vi "N5232-PNA_ReadChanTrigger.vi"(0 "Session In":refnum<visa-resource-name>="TCPIP0::169.254.70.180::inst0::INSTR", 5 "CHANNEL":i32=1, 11 "error in":errorcluster {"code" format="%.0x"}) -> (4 "Session Out":refnum<visa-resource-name>, 6 "SWE-MODE?":string, 8 "GROUP-COUNT":string, 10 "TRG-MODE":string, 15 "error out":errorcluster {"code" format="%.0x"})   [LabVIEW 2018]
doc: "Launches the Instrument I/O Assistant, which you can use to communicate with message-based instruments and graphically parse the response. For example you can communicate with an instrument that uses a serial, Ethernet, or GPIB interface."
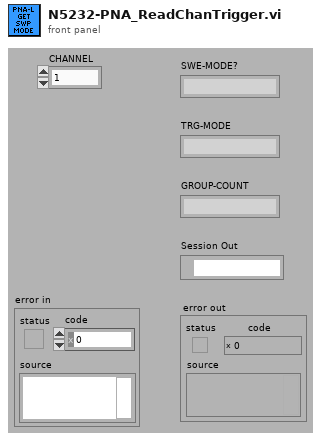
[diagram p1: front panel]
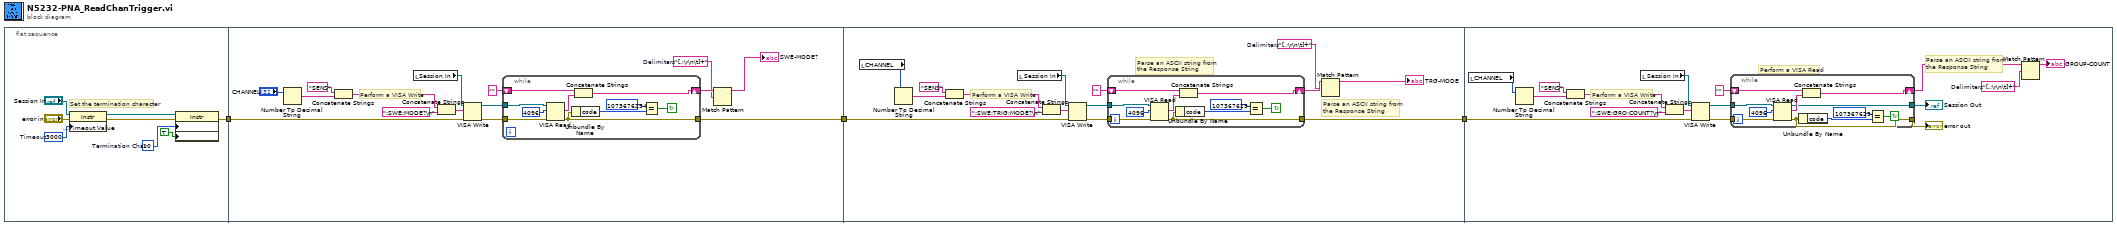
[diagram p0: block diagram]
diagram:
  n1 = flat-sequence {
    tunnel: [w7] -> w3
    tunnel: w3 -> [w17]
    tunnel: [w15] -> w2
    tunnel: w2 -> [w42]
    tunnel: [w40] -> w1
    tunnel: w1 -> [w67]
    frame #0 {
      w6 = u8 10  # Termination Char
      w10 = u32 3000  # Timeout
      # "Set the termination character"
      n2 = property class="Instr"(reference="Session In", error in="error in", "General Settings:Timeout Value"=w10) -> (reference out=w5:refnum<visa-resource-name>, error out=w8:errorcluster)
      n3 = property class="Instr"(reference=w5, error in=w8, "Message Based Settings:Termination Character"=w6, "Message Based Settings:Termination Character Enable"=TRUE ("enable")) -> (error out=w7:errorcluster)  [unwired: 1 in]
    }
    frame #1 {
      w20 = "[,;\r\n\t]+"  # Delimiters
      # "Perform a VISA Write"
      n4 = Number To Decimal String(number="CHANNEL") -> (decimal integer string=w22:string)  [unwired: 1 out]
      n5 = Concatenate Strings("SENS" ("staticText"), w22) -> (w25:string)
      n6 = local read "Session In"() -> (w14:refnum<visa-resource-name>)
      n7 = Concatenate Strings(w25, ":SWE:MODE?\n" ("StaticText")) -> (w24:string)
      n8 = VISA Write(VISA resource name=w14, write buffer=w24, error in (no error)=w17) -> (VISA resource name out=w13:refnum<visa-resource-name>, error out=w23:errorcluster)  [unwired: 1 out]
      n9 = while {
        tunnel: w13 -> [w27]
        shift-left: "" -> [w30]
        shift-right: [w29] -> w26
        tunnel: w23 -> [w28]
        tunnel: [w32] -> w15
        stop <- w34 continue-if-true
        n10 = VISA Read(VISA resource name=w27, byte count=u32 4096 ("byte count (0)"), error in (no error)=w28) -> (read buffer=w31:string, error out=w32:errorcluster)  [unwired: 2 out]
        n11 = Unbundle By Name(w32) -> ("code"=w35:i32)
        n12 = Concatenate Strings(w30, w31) -> (w29:string)
        n13 = Equal?(x=1073676294, y=w35) -> (x = y?=w34:bool)
      }
      n14 = Match Pattern(string=w26, regular expression=w20) -> (before substring=→"SWE-MODE?":string)  [unwired: 4 out]
    }
    frame #2 {
      w45 = "[,;\r\n\t]+"  # Delimiters
      # "Parse an ASCII string from the Response String"
      # "Perform a VISA Write"
      # "Parse an ASCII string from the Response String"
      n15 = local read "CHANNEL"() -> (w37:i32)
      n16 = Number To Decimal String(number=w37) -> (decimal integer string=w46:string)  [unwired: 1 out]
      n17 = Concatenate Strings("SENS" ("staticText"), w46) -> (w49:string)
      n18 = local read "Session In"() -> (w38:refnum<visa-resource-name>)
      n19 = Concatenate Strings(w49, ":SWE:TRIG:MODE?\n" ("StaticText")) -> (w48:string)
      n20 = VISA Write(VISA resource name=w38, write buffer=w48, error in (no error)=w42) -> (VISA resource name out=w39:refnum<visa-resource-name>, error out=w47:errorcluster)  [unwired: 1 out]
      n21 = while {
        shift-left: "" -> [w55]
        shift-right: [w54] -> w51
        tunnel: w47 -> [w53]
        tunnel: [w57] -> w40
        tunnel: w39 -> [w52]
        stop <- w59 continue-if-true
        n22 = VISA Read(VISA resource name=w52, byte count=u32 4096 ("byte count (0)"), error in (no error)=w53) -> (read buffer=w56:string, error out=w57:errorcluster)  [unwired: 2 out]
        n23 = Unbundle By Name(w57) -> ("code"=w60:i32)
        n24 = Concatenate Strings(w55, w56) -> (w54:string)
        n25 = Equal?(x=1073676294, y=w60) -> (x = y?=w59:bool)
      }
      n26 = Match Pattern(string=w51, regular expression=w45) -> (before substring=→"TRG-MODE":string)  [unwired: 4 out]
    }
    frame #3 {
      w70 = "[,;\r\n\t]+"  # Delimiters
      # "Parse an ASCII string from the Response String"
      # "Perform a VISA Read"
      # "Perform a VISA Write"
      n27 = local read "CHANNEL"() -> (w62:i32)
      n28 = Number To Decimal String(number=w62) -> (decimal integer string=w71:string)  [unwired: 1 out]
      n29 = Concatenate Strings("SENS" ("staticText"), w71) -> (w74:string)
      n30 = local read "Session In"() -> (w65:refnum<visa-resource-name>)
      n31 = Concatenate Strings(w74, ":SWE:GRO:COUNT?\n" ("StaticText")) -> (w73:string)
      n32 = VISA Write(VISA resource name=w65, write buffer=w73, error in (no error)=w67) -> (VISA resource name out=w64:refnum<visa-resource-name>, error out=w72:errorcluster)  [unwired: 1 out]
      n33 = while {
        shift-left: "" -> [w82]
        shift-right: [w81] -> w77
        tunnel: w72 -> [w80]
        tunnel: [w84] -> w75
        tunnel: w64 -> [w79]
        tunnel: [w78] -> w63
        stop <- w86 continue-if-true
        n34 = VISA Read(VISA resource name=w79, byte count=u32 4096 ("byte count (0)"), error in (no error)=w80) -> (VISA resource name out=w78:refnum<visa-resource-name>, read buffer=w83:string, error out=w84:errorcluster)  [unwired: 1 out]
        n35 = Unbundle By Name(w84) -> ("code"=w87:i32)
        n36 = Concatenate Strings(w82, w83) -> (w81:string)
        n37 = Equal?(x=1073676294, y=w87) -> (x = y?=w86:bool)
      }
      "error out" <- w75
      "Session Out" <- w63
      n38 = Match Pattern(string=w77, regular expression=w70) -> (before substring=→"GROUP-COUNT":string)  [unwired: 4 out]
    }
  }
